vi "9237_UI.vi"(8 "error in (no error)":errorcluster, 11 "Node Ptr":T4 format="%.0x") -> (0 "error out":errorcluster)   [LabVIEW 2017, in "Modules.lvlib" / "9237.lvclass"]
uses:
  9237.lvclass
  <vilib>/NI Veristand/Custom Device API/Custom Device Item Ref.ctl
  RSI Module/SubPanel Command.ctl
  _nicrio_cRIO-923x_ExcitationVoltageRing.ctl
  AI Settings.ctl
  Data rate.ctl
  C:/Users/dbuck/Documents/GitHub/Scan-Engine-Custom-Device-Classes/Source/RSI Module/RSI Module.lvclass
  9237.lvclass/9237.ctl
  RSI Module/RSI Module.lvclass
  <vilib>/NI Veristand/Custom Device API/Custom Device API.lvlib
panel:
  in  "ADC sampling rate":T1 items=["50.000 kS/s", "25.000 kS/s", "16.667 kS/s", "12.500 kS/s", "10.000 kS/s", "8.333 kS/s", "7.143 kS/s", "6.250 kS/s", "5.556 kS/s", "5.000 kS/s", "4.545 kS/s", "4.167 kS/s", "3.846 kS/s", "3.571 kS/s", "3.333 kS/s", "3.125 kS/s", "2.941 kS/s", "2.778 kS/s", "2.632 kS/s", "2.500 kS/s", "2.381 kS/s", "2.273 kS/s", "2.174 kS/s", "2.083 kS/s", "2.000 kS/s", "1.923 kS/s", "1.852 kS/s", "1.786 kS/s", "1.724 kS/s", "1.667 kS/s", "1.613 kS/s"]
  in  "Dynamic shunt?":bool
  in  "AI Settings":T2
  in  "Excitation Voltage":T3 items=["2.5 Volts", "3.3 Volts", "5.0 Volts", "10.0 Volts", "External Excitation"]
  in  "SubPanel Event":refnum<user-event>
  in  "Header":cluster{"Section Name":string}={"Section Name"="NI 9205 Settings"}
  # "Half-Bridge\nCompletion"
  # "Shunt Calibration\n      Enabled"
  # "AI 0"
  # "AI 1"
  # "AI 2"
  # "AI 3"
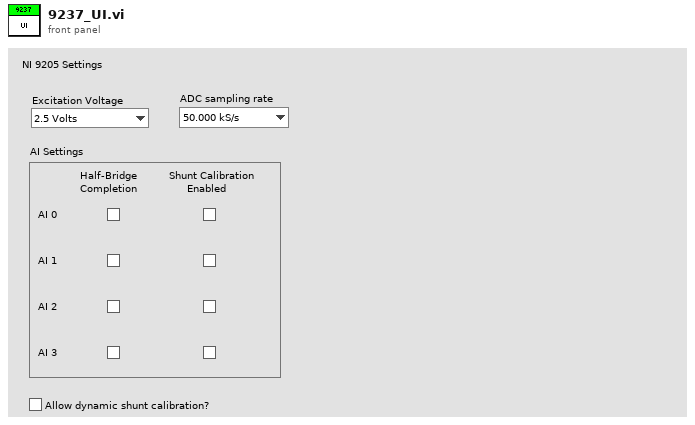
[diagram p1: front panel]
types:
  T1 = typedef "Modules.lvlib/9237.lvclass/Data rate.ctl" = u32
  T2 = typedef "Modules.lvlib/9237.lvclass/AI Settings.ctl" = cluster{"AI0 Bridge":bool, "AI0 Shunt":bool, "AI1 Bridge":bool, "AI1 Shunt":bool, "AI2 Bridge":bool, "AI2 Shunt":bool, "AI3 Bridge":bool, "AI3 Shunt":bool}
  T3 = typedef "Modules.lvlib/9237.lvclass/_nicrio_cRIO-923x_ExcitationVoltageRing.ctl" = u8
  T4 = typedef "Custom Device API.lvlib/Custom Device Item Ref.ctl" = u64
  T5 = typedef "Modules.lvlib/RSI Module.lvclass/Module Models.ctl" = enum16{"Empty", "NI 9201", "NI 9203", "NI 9205", "NI 9206", "NI 9207", "NI 9208", "NI 9211", "NI 9212", "NI 9213", "NI 9214", "NI 9215", "NI 9217", "NI 9219", "NI 9220", "NI 9221", "NI 9222", "NI 9223", "NI 9225", "NI 9227", "NI 9229", "NI 9233", "NI 9234", "NI 9235", "NI 9236", "NI 9237", "NI 9239", "NI 9242", "NI 9244", "NI 9263", "NI 9264", "NI 9265", "NI 9269", "NI 9375", "NI 9401", "NI 9402", "NI 9403", "NI 9411", "NI 9421", "NI 9422", "NI 9423", "NI 9425", "NI 9426", "NI 9435", "NI 9437", "NI 9472", "NI 9474", "NI 9475", "NI 9476", "NI 9477", "NI 9478", "NI 9481", "NI 9482", "NI 9485"}
  T6 = typedef "Modules.lvlib/RSI Module.lvclass/SubPanel Command.ctl" = enum16{"Stop"}
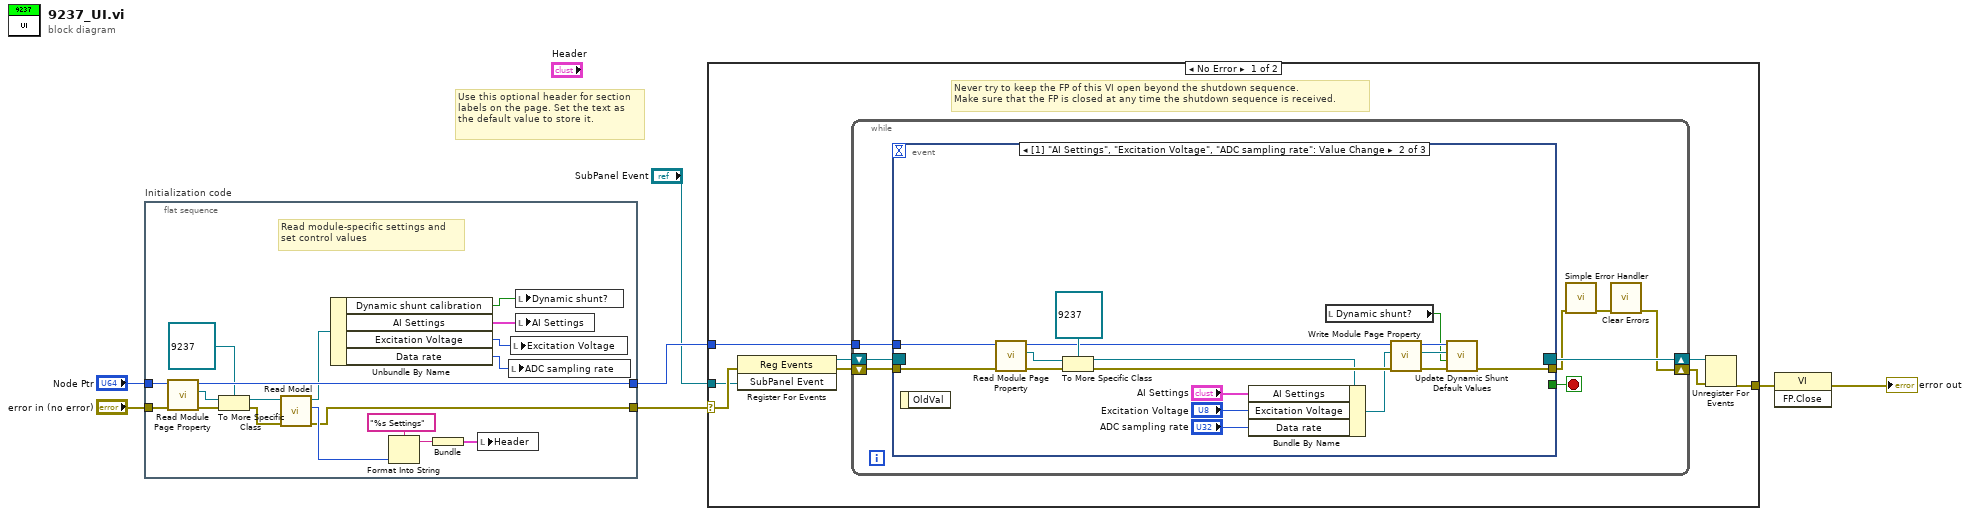
[diagram p0: block diagram]
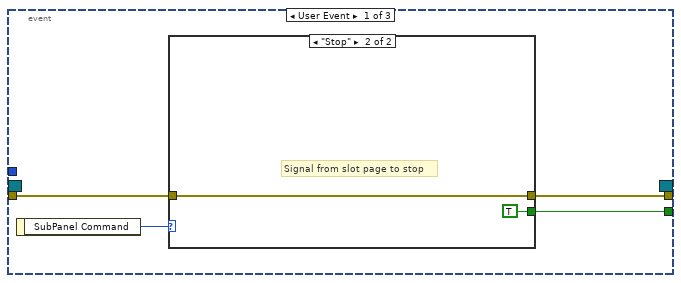
[diagram p2: hidden frame]
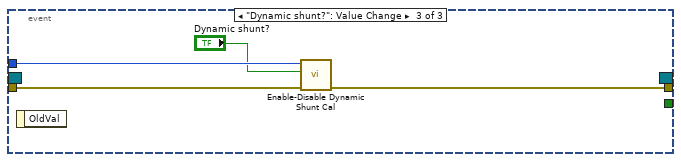
[diagram p4: hidden frame]
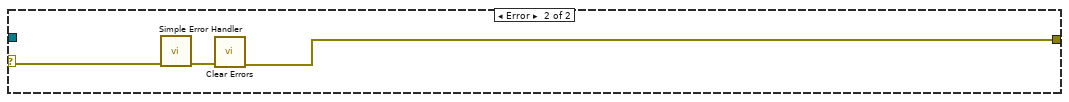
[diagram p5: hidden frame]
diagram:
  # "Use this optional header for section labels on the page. Set the text as the default value to store it."
  n1 = flat-sequence "Initialization code" {
    tunnel: "error in (no error)" -> [w24]
    tunnel: "Node Ptr" -> [w25]
    tunnel: [w12] -> w1
    tunnel: [w23] -> w4
    frame #0 {
      # "Read module-specific settings and\nset control values"
      n2 = call "Read Module Page Property.vi"("error in (no error)"=w24, "Node Ptr In"=w25) -> ("error out"=w22:errorcluster, "RSI Module"=w20:refnum<class "RSI Module.lvclass">, "Node Ptr Out"=w23:T4)  [unwired: 7 in]
      n3 = To More Specific Class(target class=refnum<class "9237.lvclass"> refnum ("9205 in"), reference=w20, error in=w22) -> (specific class reference=w19:refnum<class "9237.lvclass">, error out=w18:errorcluster)
      n4 = call "Read Model.vi"("error in (no error)"=w18, "RSI Module in"=w19) -> ("error out"=w12:errorcluster, "Model"=w16:T5, "RSI Module out"=w13:refnum<class "9237.lvclass">)  [unwired: 7 in]
      n5 = Unbundle By Name(w13) -> ("Dynamic shunt calibration"=w10:bool, "AI Settings"=w11:T2, "Excitation Voltage"=w9:T3, "Data rate"=w8:T1)
      n6 = Format Into String(format string="%s Settings", w16) -> (resulting string=w14:string)  [unwired: 2 in, 1 out]
      n7 = Bundle(w14) -> (w17:cluster{string})  [unwired: 1 in]
      n8 = local write "Header"(w17) -> ()
      n9 = local write "ADC sampling rate"(w8) -> ()
      n10 = local write "Excitation Voltage"(w9) -> ()
      n11 = local write "Dynamic shunt?"(w10) -> ()
      n12 = local write "AI Settings"(w11) -> ()
    }
  }
  n13 = case shown="No Error" w1 {
    selector: w1 -> [w27 w72]
    tunnel: [w31 w70] -> w7
    tunnel: w4 -> [w28 _]
    tunnel: "SubPanel Event" -> [w26 _]
    frame No Error {
      # "Never try to keep the FP of this VI open beyond the shutdown sequence.\nMake sure that the FP is closed at any time the shutdown sequence is received."
      n14 = register-events(error in=w27, w26) -> (reference out=w29:refnum<event-registration>, error out=w30:errorcluster)  [unwired: 1 in]
      n15 = while {
        tunnel: w28 -> [w37]
        shift-right: [w34] -> w32
        shift-left: w30 -> [w40]
        shift-right: [w41] -> w33
        shift-left: w29 -> [w39]
        stop <- w38 stop-if-true
        n16 = event shown="[1] \"AI Settings\", \"Excitation Voltage\", \"ADC sampling rate\": Value Change" {
          selector: w39 -> [_ _ _]
          dyn-events: [_ _ _] -> w41
          timeout: _ -> [_ _ _]
          tunnel: w40 -> [w44 w60 w69]
          tunnel: [w43 _ _] -> w38
          tunnel: [w42 w53 w66] -> w36
          tunnel: w37 -> [_ w61 w68]
          event User Event {
            n17 = event-data() -> ("SubPanel Command"=w45:T6)  [unwired: 1 out]
            n18 = case shown="\"Stop\"" w45 {
              tunnel: w44 -> [w46 w47]
              tunnel: [w46 w47] -> w42
              tunnel: [_ TRUE] -> w43
              frame Default {
              }
              frame "Stop" {
                # "Signal from slot page to stop"
              }
            }
          }
          event Value Change {
            n19 = event-data() -> ()  [unwired: 2 out]
            n20 = call "Read Module Page Property.vi"("error in (no error)"=w60, "Node Ptr In"=w61) -> ("error out"=w63:errorcluster, "RSI Module"=w64:refnum<class "RSI Module.lvclass">, "Node Ptr Out"=w62:T4)  [unwired: 7 in]
            n21 = To More Specific Class(target class=refnum<class "9237.lvclass"> refnum ("9205 in"), reference=w64, error in=w63) -> (specific class reference=w58:refnum<class "9237.lvclass">, error out=w59:errorcluster)
            n22 = Bundle By Name(cluster=w58, "AI Settings"="AI Settings", "Excitation Voltage"="Excitation Voltage", "Data rate"="ADC sampling rate") -> (w55:refnum<class "9237.lvclass">)
            n23 = local read "Dynamic shunt?"() -> (w50:bool)
            n24 = call "Write Module Page Property.vi"("error in (no error)"=w59, "RSI Module"=w55, "Node Ptr In"=w62) -> ("error out"=w54:errorcluster, "RSI Module out"=w52:refnum<class "9237.lvclass">, "Node Ptr Out"=w51:T4)  [unwired: 6 in]
            n25 = call "Update Dynamic Shunt Default Values.vi"("error in (no error)"=w54, "Dynamic shunt?"=w50, "9237 in"=w52, "Node Ptr in"=w51) -> ("error out"=w53:errorcluster)  [unwired: 5 in, 2 out]
          }
          event "Dynamic shunt?": Value Change {
            n26 = event-data() -> ()  [unwired: 2 out]
            n27 = call "Enable-Disable Dynamic Shunt Cal.vi"("error in"=w69, "Dynamic shunt?"="Dynamic shunt?", "Node Ptr in"=w68) -> ("error out"=w66:errorcluster)  [unwired: 7 in, 1 out]
          }
        }
        n28 = call <vilib>:"Simple Error Handler.vi"("error in (no error)"=w36) -> ("error out"=w35:errorcluster)  [unwired: 1 in, 7 out]
        n29 = call <vilib>:"Clear Errors.vi"("error in (no error)"=w35) -> ("error out"=w34:errorcluster)  [unwired: 1 in, 5 out]
      }
      n30 = Unregister For Events(event registration refnum=w33, error in=w32) -> (error out=w31:errorcluster)
    }
    frame Error {
      n31 = call <vilib>:"Simple Error Handler.vi"("error in (no error)"=w72) -> ("error out"=w71:errorcluster)  [unwired: 1 in, 7 out]
      n32 = call <vilib>:"Clear Errors.vi"("error in (no error)"=w71) -> ("error out"=w70:errorcluster)  [unwired: 1 in, 5 out]
    }
  }
  n33 = invoke class="VI" method="FP.Close"(error in=w7) -> (error out=→"error out":errorcluster)  [unwired: 2 in, 2 out]
